vi "SW_Generate_Segmented_Plot_v4_DAQmx.vi"(0 "Settings cluster in":T1={"Defaults"={"Default User"=0.0, "VISA Resource Name "="Tracker"}, "Recording and saving"={"Researcher name"="Researcher", "Name prefix"="Track", "Data filtering"=5, "Stop at"=0.0, "\"Stop at\" enabled"=FALSE}, "Geometry"={"Cage diameter, mm"=180, "Starting angle MIDFIELD"=0, "Starting angle BORDER"=0, "Radius, mm CENTER"=30, "Radius, mm MIDFIELD"=75, "N segments MIDFIELD"=2, "N segments BORDER"=4, "R-gap, mm"=0.0, "Bridge swap"=FALSE, "Bridge H. offset"=0.0, "Bridge V. offset"=0.0, "Twisted neck"=FALSE}, "IO parameters"={"SYNC configuration"=12, "IO 1 configuration"=1, "IO 2 configuration"=1, "IO 3 configuration"=0, "IO 4 configuration"=0, "Activate ext. RS-232"=0, "IO inversion config."=0}, "Stimulus presets array"=[{"Event type"=0, "Dur., s"=0.0, "Stim., s"=0.0, "TTL out N"=1, "Set/Clear"=FALSE, "Stim. has been set"=FALSE}, {"Event type"=0, "Dur., s"=0.0, "Stim., s"=0.0, "TTL out N"=1, "Set/Clear"=FALSE, "Stim. has been set"=FALSE}, {"Event type"=0, "Dur., s"=0.0, "Stim., s"=0.0, "TTL out N"=1, "Set/Clear"=FALSE, "Stim. has been set"=FALSE}, {"Event type"=0, "Dur., s"=0.0, "Stim., s"=0.0, "TTL out N"=1, "Set/Clear"=FALSE, "Stim. has been set"=FALSE}, {"Event type"=0, "Dur., s"=0.0, "Stim., s"=0.0, "TTL out N"=1, "Set/Clear"=FALSE, "Stim. has been set"=FALSE}, {"Event type"=0, "Dur., s"=0.0, "Stim., s"=0.0, "TTL out N"=1, "Set/Clear"=FALSE, "Stim. has been set"=FALSE}, {"Event type"=0, "Dur., s"=0.0, "Stim., s"=0.0, "TTL out N"=1, "Set/Clear"=FALSE, "Stim. has been set"=FALSE}, {"Event type"=0, "Dur., s"=0.0, "Stim., s"=0.0, "TTL out N"=1, "Set/Clear"=FALSE, "Stim. has been set"=FALSE}, {"Event type"=0, "Dur., s"=0.0, "Stim., s"=0.0, "TTL out N"=1, "Set/Clear"=FALSE, "Stim. has been set"=FALSE}, {"Event type"=0, "Dur., s"=0.0, "Stim., s"=0.0, "TTL out N"=1, "Set/Clear"=FALSE, "Stim. has been set"=FALSE}, {"Event type"=0, "Dur., s"=0.0, "Stim., s"=0.0, "TTL out N"=1, "Set/Clear"=FALSE, "Stim. has been set"=FALSE}, {"Event type"=0, "Dur., s"=0.0, "Stim., s"=0.0, "TTL out N"=1, "Set/Clear"=FALSE, "Stim. has been set"=FALSE}, {"Event type"=0, "Dur., s"=0.0, "Stim., s"=0.0, "TTL out N"=1, "Set/Clear"=FALSE, "Stim. has been set"=FALSE}, {"Event type"=0, "Dur., s"=0.0, "Stim., s"=0.0, "TTL out N"=1, "Set/Clear"=FALSE, "Stim. has been set"=FALSE}], "Settings loaded OK"=FALSE} {"Stimulus presets array"."Event type" items=["Stay for N seconds"]; "Stimulus presets array"."TTL out N" items=["1"=1, "2"=2, "1+2"=3]; "Geometry"."Cage diameter, mm" scale=0.0..340.0}, 1 "Regions to mark set (none)":u16[](array[numeric]), 2 "Regions to mark selected (none)":u16[](array[numeric]), 5 "Draw Area Size (480x480)":T5={"Width"=480, "Height"=480}, 7 "Scale factor for outer display radius display (0.95)":dbl=0.95 format="%#_13g", 9 "Segments Colors In":T3={"Colors array for outer segments"=[14102567, 16625249, 14742520, 7646673, 16018755, 16703632, 11262441, 4552116], "Colors array for midfield segments"=[8073876, 10935200, 34871, 12756431], "Color for central segment"=16777113, "Fill color for no segments image"=6316128}, 11 "Error In":errorcluster, 12 "Show magnets (T)":bool=TRUE, 13 "Show zones (T)":bool=TRUE) -> (4 "Experiment Diagram":T4(plugin-control), 6 "Array of the pixel to color correspondences":u32[][](array[numeric]), 8 "Array of the segment to color correspondences":u32[][](array[numeric]), 10 "Settings cluster out":T1={"Defaults"={"Default User"=0.0, "VISA Resource Name "="Tracker"}, "Recording and saving"={"Researcher name"="Researcher", "Name prefix"="Track", "Data filtering"=5, "Stop at"=0.0, "\"Stop at\" enabled"=FALSE}, "Geometry"={"Cage diameter, mm"=180, "Starting angle MIDFIELD"=0, "Starting angle BORDER"=0, "Radius, mm CENTER"=30, "Radius, mm MIDFIELD"=75, "N segments MIDFIELD"=2, "N segments BORDER"=4, "R-gap, mm"=0.0, "Bridge swap"=FALSE, "Bridge H. offset"=0.0, "Bridge V. offset"=0.0, "Twisted neck"=FALSE}, "IO parameters"={"SYNC configuration"=12, "IO 1 configuration"=1, "IO 2 configuration"=1, "IO 3 configuration"=0, "IO 4 configuration"=0, "Activate ext. RS-232"=0, "IO inversion config."=0}, "Stimulus presets array"=[{"Event type"=0, "Dur., s"=0.0, "Stim., s"=0.0, "TTL out N"=1, "Set/Clear"=FALSE, "Stim. has been set"=FALSE}, {"Event type"=0, "Dur., s"=0.0, "Stim., s"=0.0, "TTL out N"=1, "Set/Clear"=FALSE, "Stim. has been set"=FALSE}, {"Event type"=0, "Dur., s"=0.0, "Stim., s"=0.0, "TTL out N"=1, "Set/Clear"=FALSE, "Stim. has been set"=FALSE}, {"Event type"=0, "Dur., s"=0.0, "Stim., s"=0.0, "TTL out N"=1, "Set/Clear"=FALSE, "Stim. has been set"=FALSE}, {"Event type"=0, "Dur., s"=0.0, "Stim., s"=0.0, "TTL out N"=1, "Set/Clear"=FALSE, "Stim. has been set"=FALSE}, {"Event type"=0, "Dur., s"=0.0, "Stim., s"=0.0, "TTL out N"=1, "Set/Clear"=FALSE, "Stim. has been set"=FALSE}, {"Event type"=0, "Dur., s"=0.0, "Stim., s"=0.0, "TTL out N"=1, "Set/Clear"=FALSE, "Stim. has been set"=FALSE}, {"Event type"=0, "Dur., s"=0.0, "Stim., s"=0.0, "TTL out N"=1, "Set/Clear"=FALSE, "Stim. has been set"=FALSE}, {"Event type"=0, "Dur., s"=0.0, "Stim., s"=0.0, "TTL out N"=1, "Set/Clear"=FALSE, "Stim. has been set"=FALSE}, {"Event type"=0, "Dur., s"=0.0, "Stim., s"=0.0, "TTL out N"=1, "Set/Clear"=FALSE, "Stim. has been set"=FALSE}, {"Event type"=0, "Dur., s"=0.0, "Stim., s"=0.0, "TTL out N"=1, "Set/Clear"=FALSE, "Stim. has been set"=FALSE}, {"Event type"=0, "Dur., s"=0.0, "Stim., s"=0.0, "TTL out N"=1, "Set/Clear"=FALSE, "Stim. has been set"=FALSE}, {"Event type"=0, "Dur., s"=0.0, "Stim., s"=0.0, "TTL out N"=1, "Set/Clear"=FALSE, "Stim. has been set"=FALSE}, {"Event type"=0, "Dur., s"=0.0, "Stim., s"=0.0, "TTL out N"=1, "Set/Clear"=FALSE, "Stim. has been set"=FALSE}], "Settings loaded OK"=FALSE} {"Stimulus presets array"."Event type" items=["Stay for N seconds"]; "Stimulus presets array"."TTL out N" items=["1"=1, "2"=2, "1+2"=3]; "Geometry"."Cage diameter, mm" scale=0.0..340.0}, 15 "Error Out":errorcluster)   [LabVIEW 2018]
uses:
  Controls/CTL_Draw_Area_Size.ctl
  Controls/CTL_Settings_cluster.ctl
  Controls/CTL_Single_stimulus_setting.ctl
panel:
  in  "Background color":u32(colorbox)=13816530
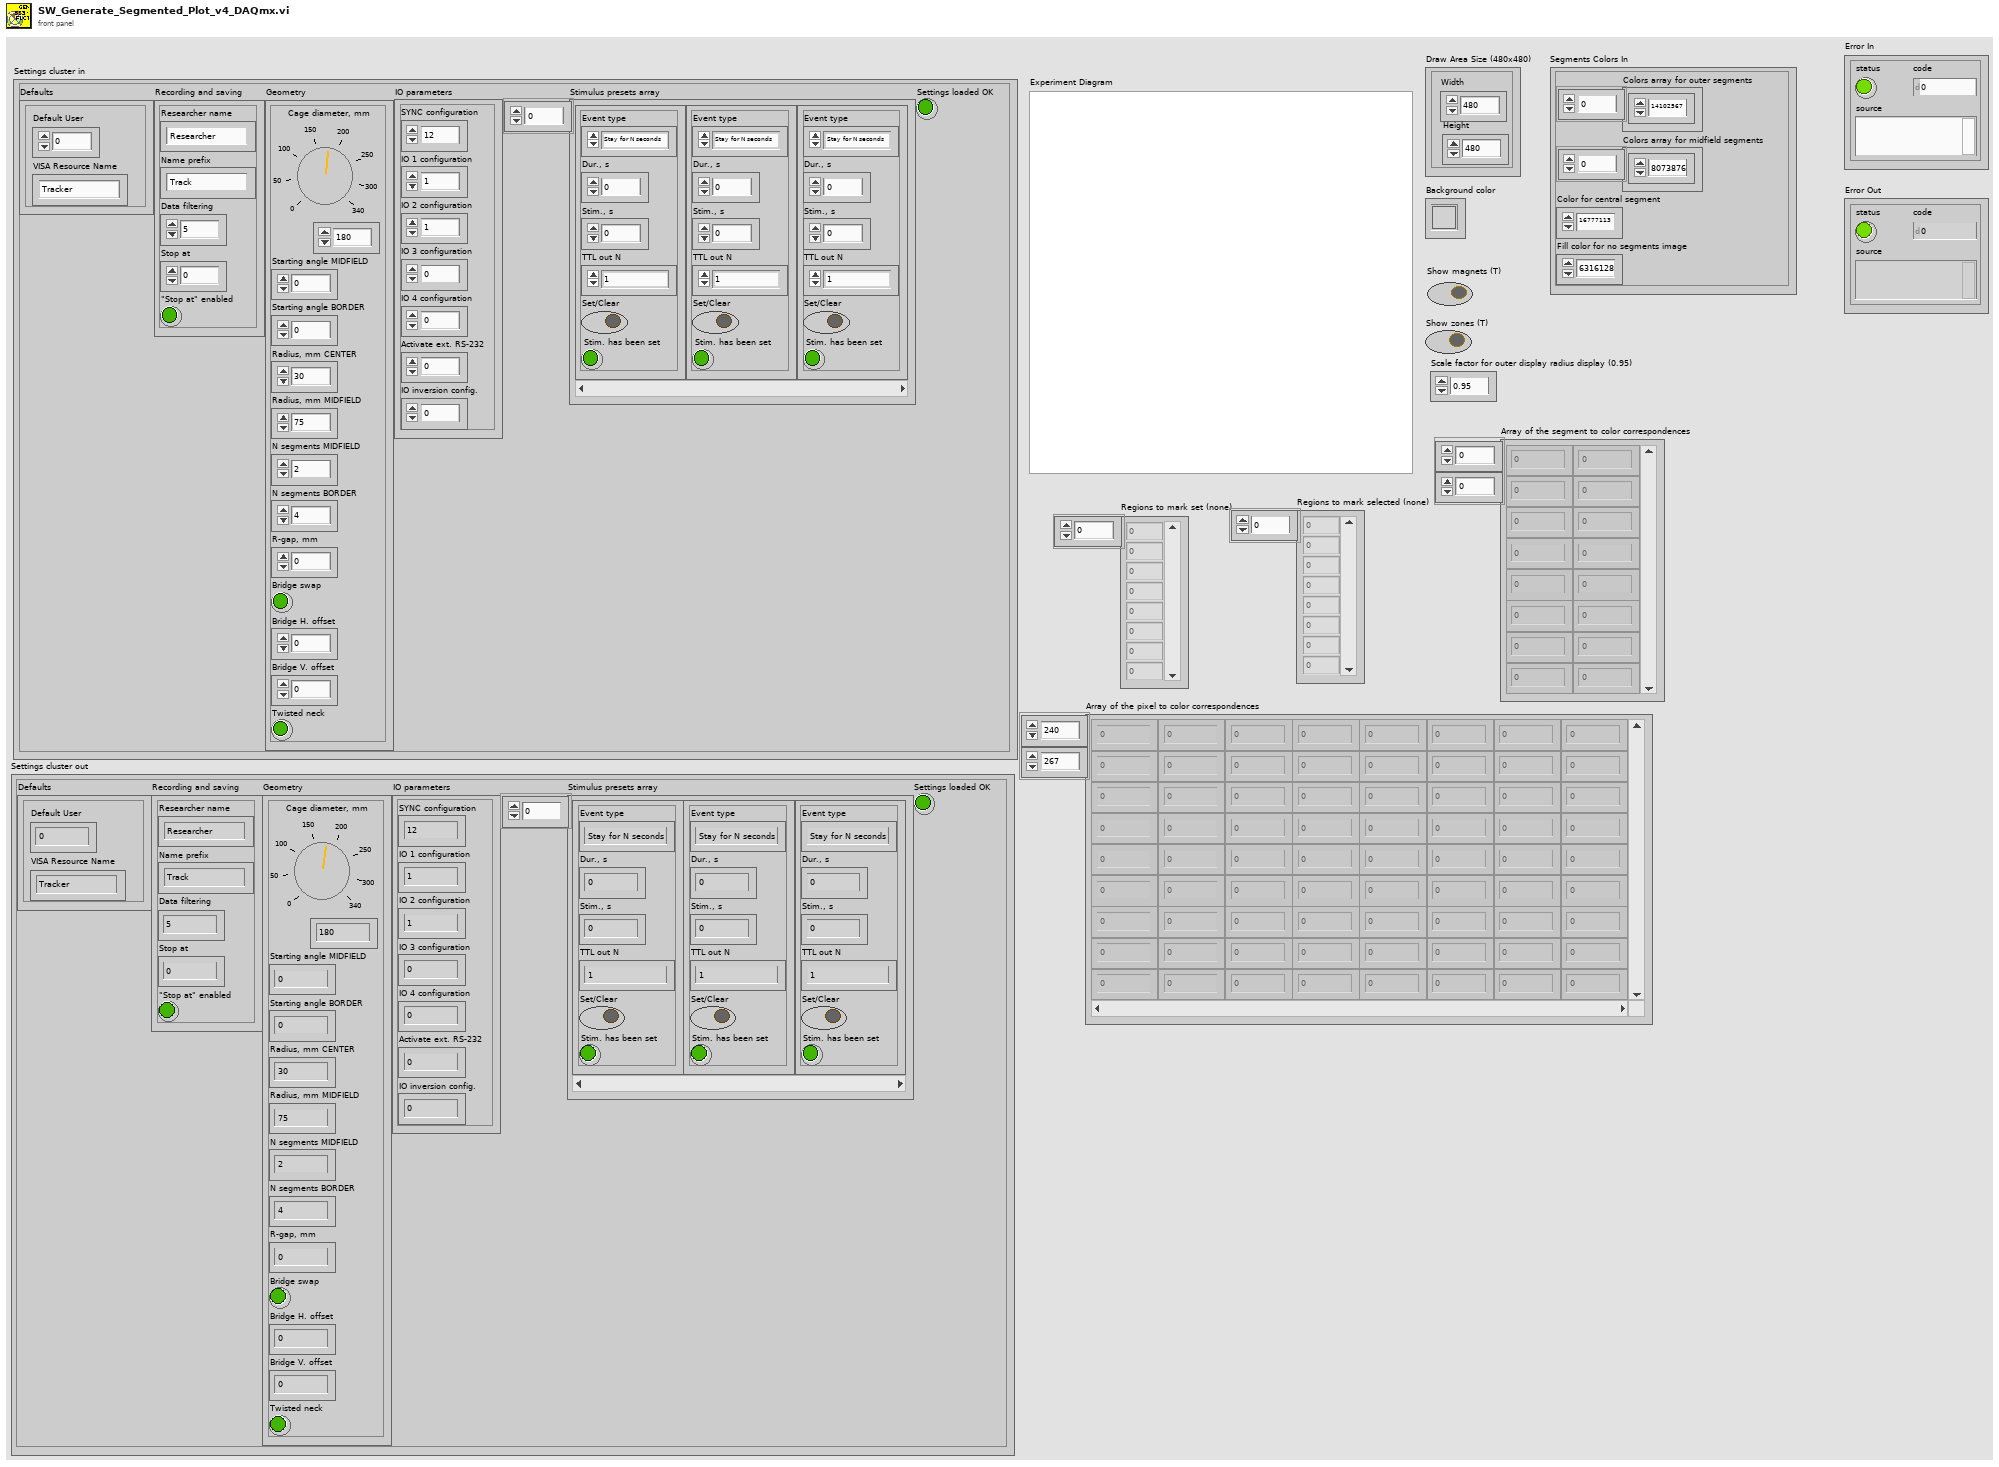
[diagram p1: front panel]
types:
  T1 = typedef "CTL_Settings_cluster.ctl" = cluster{"Defaults":cluster{"Default User":dbl, "VISA Resource Name ":string}, "Recording and saving":cluster{"Researcher name":string, "Name prefix":string, "Data filtering":u16, "Stop at":dbl, "\"Stop at\" enabled":bool}, "Geometry":cluster{"Cage diameter, mm":u16, "Starting angle MIDFIELD":i16, "Starting angle BORDER":i16, "Radius, mm CENTER":u16, "Radius, mm MIDFIELD":u16, "N segments MIDFIELD":u8, "N segments BORDER":u8, "R-gap, mm":sgl, "Bridge swap":bool, "Bridge H. offset":sgl, "Bridge V. offset":sgl, "Twisted neck":bool}, "IO parameters":cluster{"SYNC configuration":u16, "IO 1 configuration":u16, "IO 2 configuration":u16, "IO 3 configuration":u16, "IO 4 configuration":u16, "Activate ext. RS-232":u16, "IO inversion config.":u16}, "Stimulus presets array":T2[], "Settings loaded OK":bool}
  T2 = typedef "CTL_Single_stimulus_setting.ctl" = cluster{"Event type":u16, "Dur., s":sgl, "Stim., s":sgl, "TTL out N":u16, "Set/Clear":bool, "Stim. has been set":bool}
  T3 = cluster{"Colors array for outer segments":u32[], "Colors array for midfield segments":u32[], "Color for central segment":u32, "Fill color for no segments image":u32}
  T4 = typedef "IMAQ Image.ctl" = refnum<image>
  T5 = typedef "CTL_Draw_Area_Size.ctl" = cluster{"Width":i32, "Height":i32}
  T6 = cluster{"Cage diameter, mm":u16, "Starting angle MIDFIELD":i16, "Starting angle BORDER":i16, "Radius, mm CENTER":u16, "Radius, mm MIDFIELD":u16, "N segments MIDFIELD":u8, "N segments BORDER":u8, "R-gap, mm":sgl, "Bridge swap":bool, "Bridge H. offset":sgl, "Bridge V. offset":sgl, "Twisted neck":bool}
  T7 = typedef "CTL_Image_Geometrical_and_scaling_parameters.ctl" = cluster{"Fonts scale factor":dbl, "Pixels per mm":dbl, "Radius of displayed outer segments, pix":dbl, "Radius of displayed midfield segments, pix":dbl, "Radius of displayed central segment, pix":dbl}
  T8 = typedef "CTL_Bounding_Rectangle_of_Segments.ctl" = cluster{"Bounding rectangle for outer segments, pix":cluster{"TL W, pix":i32, "TL H, pix":i32, "RB W, pix":i32, "RB H, pix":i32}, "Bounding rectangle of the midfield segments, pix":cluster{"TL W, pix":i32, "TL H, pix":i32, "RB W, pix":i32, "RB H, pix":i32}, "Coordinates of the center of the image, pix":cluster{"W, pix":i32, "H, pix":i32}, "Bounding rectangle of the central segment, pix":cluster{"Numeric Control":i32, "Numeric Control":i32, "Numeric Control":i32, "Numeric Control":i32}}
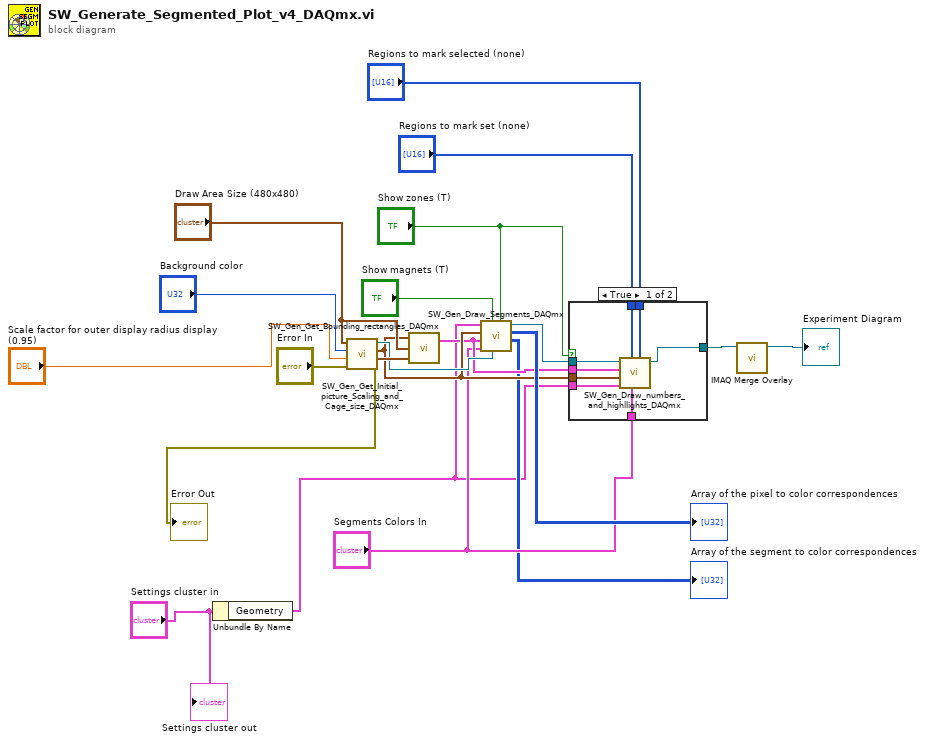
[diagram p0: block diagram]
diagram:
  n1 = Unbundle By Name("Settings cluster in") -> ("Geometry"=w1:T6)
  n2 = call "SW_Gen_Get_Initial_picture_Scaling_and_Cage_size_DAQmx.vi"("Error In"="Error In", "Scale factor for outer display radius display"="Scale factor for outer display radius display (0.95)", "Background color"="Background color", "Draw Area Size"="Draw Area Size (480x480)") -> ("Error Out"=→"Error Out":errorcluster, "Width of the borders combined out"=w14:cluster{"Width":i32, "Height":i32}, "Image geometrical and scaling parameters"=w11:T7, "Background Image"=w13:T4)  [unwired: 4 in]
  n3 = call "SW_Gen_Get_Bounding_rectangles_DAQmx.vi"("Width of the borders combined"=w14, "Draw Area Size"="Draw Area Size (480x480)", "Image geometrical and scaling parameters"=w11) -> ("Bounding rectangles"=w10:T8)  [unwired: 1 in]
  n4 = call "SW_Gen_Draw_Segments_DAQmx.vi"("Show zones"="Show zones (T)", "Cage Image ref"=w13, "Show magnets"="Show magnets (T)", "Colors cluster"="Segments Colors In", "Bounding rectangles"=w10, "Image geometrical and scaling parameters"=w11, "Input cluster of parameters"=w1) -> ("Array of the segment to color correspondences"=→"Array of the segment to color correspondences":u32[][], "Array of the pixel to color correspondences"=→"Array of the pixel to color correspondences":u32[][], "Cage Image out"=w8:T4)  [unwired: 2 in]
  n5 = case shown="True" "Show zones (T)" {
    tunnel: "Regions to mark set (none)" -> [w29 _]
    tunnel: "Regions to mark selected (none)" -> [w28 _]
    tunnel: w11 -> [w27 _]
    tunnel: w10 -> [w26 _]
    tunnel: "Segments Colors In" -> [w25 _]
    tunnel: w1 -> [w24 _]
    tunnel: w8 -> [w23 w30]
    tunnel: [w22 w30] -> w3
    frame True {
      n6 = call "SW_Gen_Draw_numbers_and_highllights_DAQmx.vi"("Regions to mark selected"=w28, "Colors cluster"=w25, "Regions to mark set"=w29, "Input cluster of parameters"=w24, "Image geometrical and scaling parameters"=w27, "Bounding rectangles"=w26, "Experiment Diagram"=w23) -> ("Experiment Diagram out"=w22:T4)  [unwired: 4 in]
    }
    frame False {
    }
  }
  n7 = call "IMAQ Merge Overlay"("Image Src"=w3) -> ("Image Dst Out"=→"Experiment Diagram":T4)  [unwired: 9 in, 1 out]
  "Settings cluster out" <- "Settings cluster in"
